vi "GetSystemHealth.vi"(7 "LabVIEW Web Service Request":refnum<class "Web Request.lvclass">) -> ()   [LabVIEW 2017]
uses:
  <vilib>/wsapi/Web Request.lvclass
  <vilib>/addons/SystemInfoProcess/SystemInfoProcess.lvlib
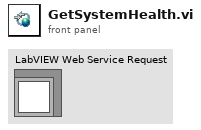
[diagram p1: front panel]
types:
  T1 = typedef "PointValueMap.lvlib/PointMap.ctl" = refnum<data-value>
  T2 = typedef "SystemInfoProcess.lvlib/SystemResources.ctl" = cluster{"TotalPhysicalMemory":dbl, "FreePhysicalMemory":dbl, "LargestAvailableMemoryBlock":dbl, "TotalVirtualMemory":dbl, "FreeVirtualMemory":dbl, "PrimaryDiskCapacity":dbl, "PrimaryDiskFree":dbl, "Utilization":T3, "CPU Loads":T4[]}
  T3 = typedef "SystemInfoProcess.lvlib/Utilization.ctl" = cluster{"CPU":dbl, "Memory":dbl, "Disk":dbl}
  T4 = typedef "SystemInfoProcess.lvlib/CPULoad.ctl" = cluster{"Total (%)":dbl, "Time Critical (%)":dbl, "Timed Structures (%)":dbl, "High (%)":dbl, "Above Normal (%)":dbl, "Normal (%)":dbl, "Background (%)":dbl, "Idle (%)":dbl, "ISR (%)":dbl}
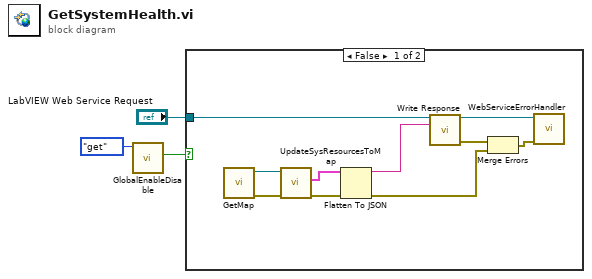
[diagram p0: block diagram]
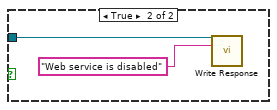
[diagram p2: hidden frame]
diagram:
  n1 = call "GlobalEnableDisable.vi"("action"=enum16{"init", "set", "get"}."get") -> ("DisableDeviceWebService"=w1:bool)  [unwired: 10 in]
  n2 = case shown="False" w1 {
    tunnel: "LabVIEW Web Service Request" -> [w13 w14]
    frame False {
      n3 = call <vilib>:"GetMap.vi"() -> ("error out"=w9:errorcluster, "SystemInfoMap"=w8:T1)  [unwired: 10 in]
      n4 = call <vilib>:"UpdateSysResourcesToMap.vi"("error in (no error)"=w9, "map in"=w8) -> ("error out"=w5:errorcluster, "system resources"=w7:T2)  [unwired: 7 in, 1 out]
      n5 = Flatten To JSON(anything=w7, error in (no error)=w5) -> (JSON string=w6:string, 11:w4:errorcluster)  [unwired: 1 in]
      n6 = call <vilib>:"Write Response.vi"("LabVIEW Web Service Request"=w13, "response string"=w6) -> ("LabVIEW Web Service Request out"=w12:refnum<class "Web Request.lvclass">, "error out"=w11:errorcluster)  [unwired: 12 in]
      n7 = Merge Errors(w11, w4) -> (w10:errorcluster)
      n8 = call "WebServiceErrorHandler.vi"("LabVIEW Web Service Request"=w12, "error in (no error)"=w10) -> ()  [unwired: 12 in, 2 out]
    }
    frame True {
      n9 = call <vilib>:"Write Response.vi"("LabVIEW Web Service Request"=w14, "response string"="Web service is disabled") -> ()  [unwired: 12 in, 2 out]
    }
  }
